vi "RT Driver VI.vi"(7 "Operation":T1, 11 "Device Reference in":T2 format="%.0x") -> (0 "Error Code":i32)   [LabVIEW 2026, in "WebPage Addon Engine.lvlib"]
uses:
  WebPage Addon Engine.lvlib
  <vilib>/NI VeriStand/Custom Device API/Custom Device Item Ref.ctl
  <vilib>/NI VeriStand/Custom Device API/Hardware Interface Driver VI Operation.ctl
  <vilib>/NI/NIVS Inline Async API/_VS Inline Async API/VS Inline Async API/VS Inline Async API.lvclass
  Addon Shared/Types/Compiled.Settings.ctl
  <vilib>/NI/NIVS Inline Async API/_VS Inline Async API/VS Inline Async API/VS Inline Async API.lvclass/VS Inline Async API.ctl
  <vilib>/NI/NIVS Inline Async API/_Data Access Engine/Data Access Engine/Data Access Engine.lvclass/Data Access Engine.ctl
  <vilib>/NI/NIVS Inline Async API/_Data Access Engine/Access Type Classes/Write/Write.lvclass/Write.ctl
  <vilib>/NI/NIVS Inline Async API/_Data Access Engine/Access Type Classes/ReadWrite/ReadWrite.lvclass/ReadWrite.ctl
  <vilib>/NI/NIVS Inline Async API/_Data Access Engine/Access Type Classes/Read/Read.lvclass/Read.ctl
  <vilib>/NI/NIVS Inline Async API/_Data Access Engine/Data Access Engine/Methods/Data.Engine.Read Data from HW.vi
  <vilib>/NI/NIVS Inline Async API/_VS Inline Async API/Error Handling Process/SubVIs/Error.GetError.vi
  <vilib>/NI/NIVS Inline Async API/_Data Access Engine/Data Access Engine/Methods/Data.Engine.Write Data to HW.vi
  <vilib>/NI/NIVS Inline Async API/_Data Access Engine/Access Type Classes/ReadWrite/ReadWrite.EngineData.vi
  <vilib>/NI/NIVS Inline Async API/_Data Access Engine/Access Type Classes/Write/Write.EngineData.vi
  <vilib>/NI/NIVS Inline Async API/_Data Access Engine/Access Type Classes/Read/Read.EngineData.vi
  <vilib>/NI VeriStand/Custom Device API/NI VeriStand - Get Channel Value by Data Reference.vi
  <vilib>/NI VeriStand/Custom Device API/NI VeriStand - Set Channel Value by Data Reference.vi
  <vilib>/NI VeriStand/Custom Device API/NI VeriStand - Set Channel Values by Block Data Reference.vi
  <vilib>/NI VeriStand/Custom Device API/NI VeriStand - Get Channel Values by Block Data Reference.vi
  Addon Shared/Constants.vi
  WebPage Addon.Async.vi
  <vilib>/Utility/SystemLogging/Write to System Log.vi
  <vilib>/NI VeriStand/Custom Device API/Get Item Property (Variant).vi
  <vilib>/NI VeriStand/Custom Device API/Global Data Refs.vi
  <vilib>/NI VeriStand/Custom Device API/Custom Device API.lvlib
  Addon Shared/WebPage Addon Shared.lvlib
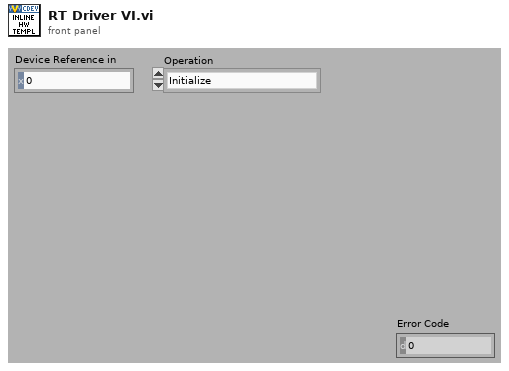
[diagram p1: front panel]
types:
  T1 = typedef "Custom Device API.lvlib/Hardware Interface Driver VI Operation.ctl" = enum16{"Initialize", "Start", "Read Data from HW", "Write Data to HW", "Close"}
  T2 = typedef "Custom Device API.lvlib/Custom Device Item Ref.ctl" = u64
  T3 = typedef "WebPage Addon Shared.lvlib/Compiled.Settings.ctl" = cluster{"Name":string, "Decimation":u32, "Channel Names":string[], "Hosted IP Address":string, "Hosted Port":u32, "gRPC Port":u32}
  T4 = cluster{"Async":refnum<class "VS Inline Async API.lvclass">, "Settings":T3, "Iteration Count":i32}
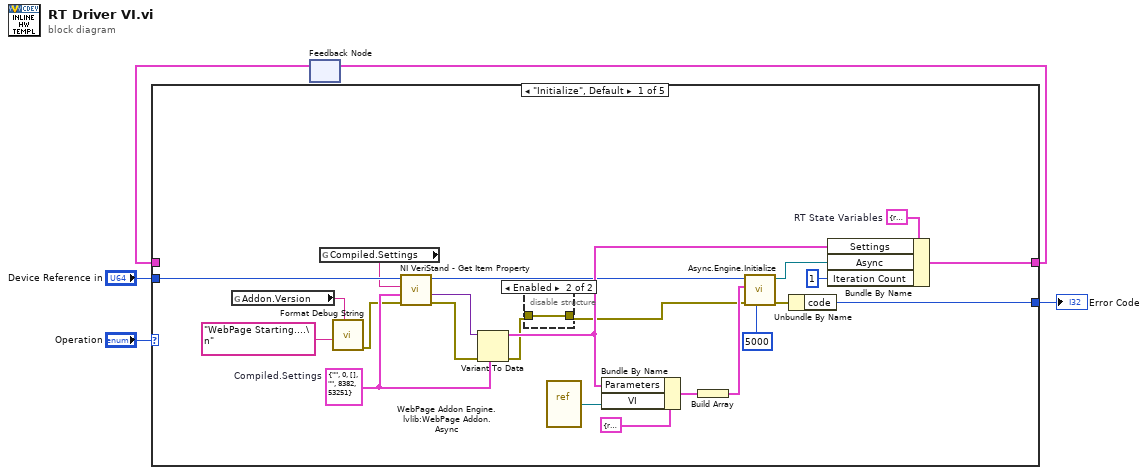
[diagram p0: block diagram]
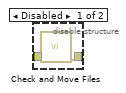
[diagram p2: hidden frame]
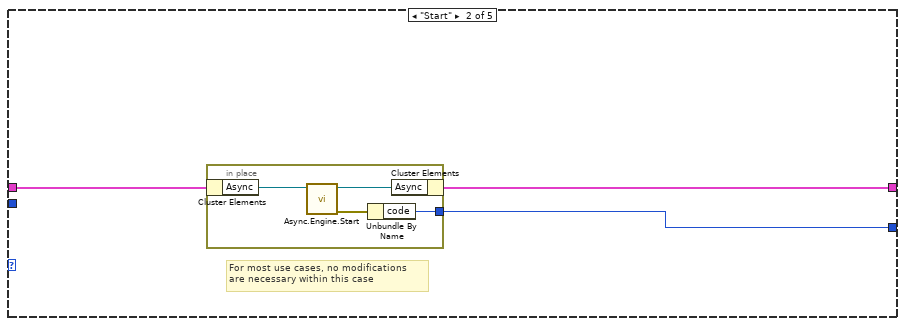
[diagram p3: hidden frame]
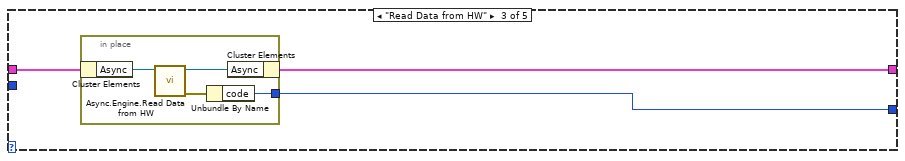
[diagram p4: hidden frame]
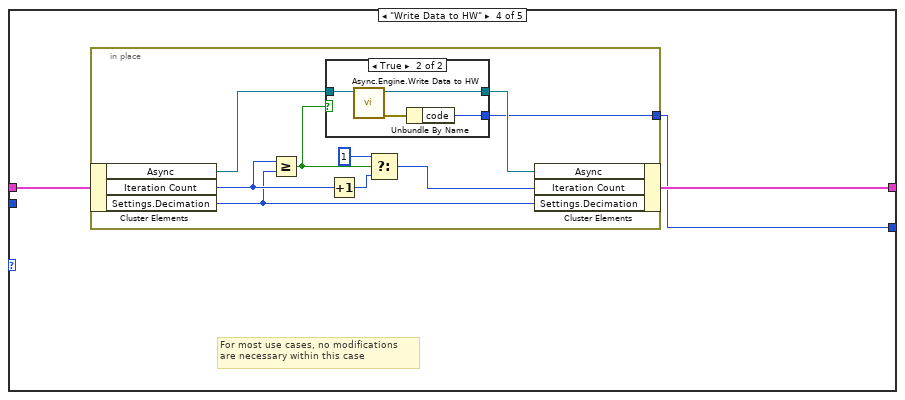
[diagram p5: hidden frame]
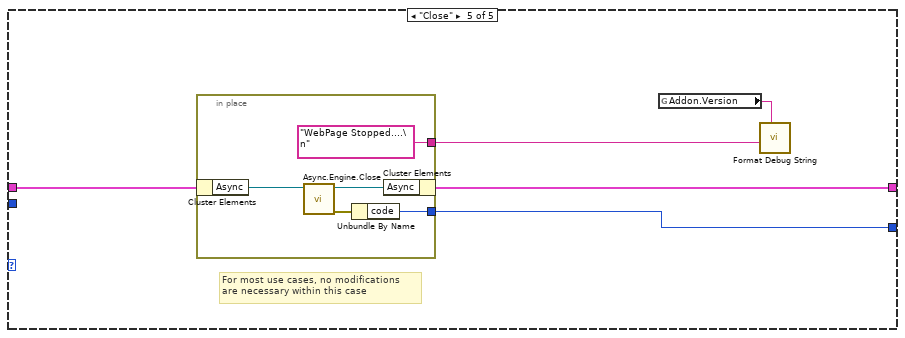
[diagram p7: hidden frame]
diagram:
  n1 = feedback #1() -> (w3:T4)  [unwired: 1 out]
  n2 = case shown="\"Initialize\", Default" "Operation" {
    tunnel: [w26 w33 w39 w47 w66] -> w4
    tunnel: w3 -> [_ w34 w40 w48 w67]
    tunnel: "Device Reference in" -> [w23 _ _ _ _]
    tunnel: [w28 w32 w41 w46 w65] -> w1
    frame "Initialize", Default {
      w18 = T4 {"Async"=refnum, "Settings"={"Name"="", "Decimation"=0, "Channel Names"=[], "Hosted IP Address"="", "Hosted Port"=8382, "gRPC Port"=53251}, "Iteration Count"=0}  # RT State Variables
      w19 = T3 {"Name"="", "Decimation"=0, "Channel Names"=[], "Hosted IP Address"="", "Hosted Port"=8382, "gRPC Port"=53251}  # Compiled.Settings
      n3 = global read "Constants.vi" "Addon.Version"() -> (w10:string)
      n4 = global read "Constants.vi" "Compiled.Settings"() -> (w20:string)
      n5 = call "Format Debug String.vi"("Version"=w10, "State"="WebPage Starting....\n") -> ("error out"=w8:errorcluster)  [unwired: 9 in]
      n6 = call-poly <vilib>:"NI VeriStand - Get Item Property.vi"("error in (no error)"=w8, "Default Value"=w19, "Property Name"=w20, "Item Ref in"=w23) -> ("error out"=w22:errorcluster, "Value"=w21:variant, "Item Ref out"=w13:T2)  [unwired: 4 in, 1 out]
      n7 = Variant To Data(error in=w22, type=w19, Variant=w21) -> (data=w15:T3, error out=w7:errorcluster)
      n8 = disable-structure shown="Enabled" {
        disable-tunnel: w7 -> [w30 w31]
        disable-tunnel: [w29 w31] -> w6
        frame Disabled {
          n9 = call "Check and Move Files.vi"("error in"=w30) -> ("error out"=w29:errorcluster)  [unwired: 10 in]
        }
        frame Enabled {
        }
      }
      n10 = vi-ref "WebPage Addon Engine.lvlib:WebPage Addon.Async.vi"() -> (w16:refnum<vi>)
      n11 = Bundle By Name(cluster=cluster{"VI":refnum<vi>, "Parameters":variant} {"VI"=refnum, "Parameters"=variant} ("Process"), "Parameters"=w15, "VI"=w16) -> (w24:cluster{"VI":refnum<vi>, "Parameters":variant})
      n12 = Build Array(w24) -> (w17:cluster{"VI":refnum<vi>, "Parameters":variant}[])
      n13 = call <vilib>:"Async.Engine.Initialize.vi"("Timeout (ms) (5000)"=u16 5000, "error in (no error)"=w6, "Processes"=w17, "Custom Device Ref"=w13) -> ("error out"=w14:errorcluster, "Async"=w27:refnum<class "VS Inline Async API.lvclass">)  [unwired: 6 in]
      n14 = Unbundle By Name(w14) -> ("code"=w28:i32)
      n15 = Bundle By Name(cluster=w18, "Settings"=w15, "Async"=w27, "Iteration Count"=1) -> (w26:T4)
    }
    frame "Start" {
      # "For most use cases, no modifications \nare necessary within this case"
      n16 = in-place {
        in-place-border: [w35] -> w32
        n17 = in-place-cluster #2(w34) -> ("Async"=w38:refnum<class "VS Inline Async API.lvclass">)
        n18 = call <vilib>:"Async.Engine.Start.vi"("VS Inline Async API in"=w38) -> ("error out"=w36:errorcluster, "VS Inline Async API out"=w37:refnum<class "VS Inline Async API.lvclass">)  [unwired: 9 in]
        n19 = Unbundle By Name(w36) -> ("code"=w35:i32)
        n20 = in-place-cluster #2("Async"=w37) -> (w33:T4)
      }
    }
    frame "Read Data from HW" {
      n21 = in-place {
        in-place-border: [w45] -> w41
        n22 = in-place-cluster #3(w40) -> ("Async"=w43:refnum<class "VS Inline Async API.lvclass">)
        n23 = call <vilib>:"Async.Engine.Read Data from HW.vi"("Async in"=w43) -> ("error out"=w44:errorcluster, "Async out"=w42:refnum<class "VS Inline Async API.lvclass">)  [unwired: 9 in]
        n24 = Unbundle By Name(w44) -> ("code"=w45:i32)
        n25 = in-place-cluster #3("Async"=w42) -> (w39:T4)
      }
    }
    frame "Write Data to HW" {
      # "For most use cases, no modifications \nare necessary within this case"
      n26 = in-place {
        in-place-border: [w55] -> w46
        n27 = in-place-cluster #4(w48) -> ("Async"=w57:refnum<class "VS Inline Async API.lvclass">, "Iteration Count"=w52:i32, "Settings.Decimation"=w49:u32)
        n28 = Greater Or Equal?(x=w52, y=w49) -> (x >= y?=w54:bool)
        n29 = case shown="True" w54 {
          tunnel: w57 -> [w58 w61]
          tunnel: [w58 w59] -> w56
          tunnel: [_ w62] -> w55
          frame False {
          }
          frame True {
            n30 = call <vilib>:"Async.Engine.Write Data to HW.vi"("VS Inline Async API in"=w61) -> ("error out"=w60:errorcluster, "VS Inline Async API out"=w59:refnum<class "VS Inline Async API.lvclass">)  [unwired: 9 in]
            n31 = Unbundle By Name(w60) -> ("code"=w62:i32)
          }
        }
        n32 = Increment(x=w52) -> (x+1=w51:i32)
        n33 = Select(t=1 ("Iteration Count"), s=w54, f=w51) -> (s? t:f=w50:i32)
        n34 = in-place-cluster #4("Async"=w56, "Iteration Count"=w50, "Settings.Decimation"=w49) -> (w47:T4)
      }
    }
    frame "Close" {
      # "For most use cases, no modifications \nare necessary within this case"
      n35 = in-place {
        in-place-border: [w70] -> w65
        in-place-border: ["WebPage Stopped....\n" ("State")] -> w63
        n36 = in-place-cluster #5(w67) -> ("Async"=w72:refnum<class "VS Inline Async API.lvclass">)
        n37 = call <vilib>:"Async.Engine.Close.vi"("Async in"=w72) -> ("error out"=w69:errorcluster, "Async out"=w71:refnum<class "VS Inline Async API.lvclass">)  [unwired: 9 in]
        n38 = Unbundle By Name(w69) -> ("code"=w70:i32)
        n39 = in-place-cluster #5("Async"=w71) -> (w66:T4)
      }
      n40 = global read "Constants.vi" "Addon.Version"() -> (w64:string)
      n41 = call "Format Debug String.vi"("Version"=w64, "State"=w63) -> ()  [unwired: 9 in, 1 out]
    }
  }
  "Error Code" <- w1
  n42 = feedback-in #1(w4) -> ()
